vi "TDT ET-Send Command.vi"(0 "TCP":T1, 2 "Command":T2, 7 "Param (int)":i32, 9 "Timeout (ms)":i32=5000, 11 "error in (no error)":errorcluster) -> (4 "TCP Thru":T1, 10 "Return Value":i32, 15 "error out":errorcluster)   [LabVIEW 2020]
uses:
  Utility VIs/Type Defs/TCP Params.ctl
  TDT ET-Command Enum.ctl
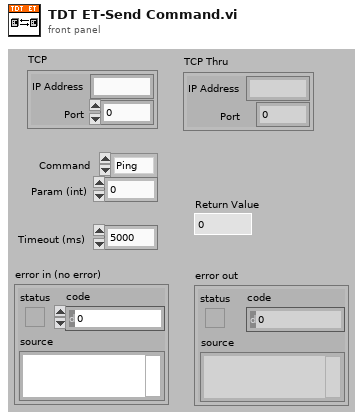
[diagram p1: front panel]
types:
  T1 = typedef "TCP Params.ctl" = cluster{"IP Address":string, "Port":i32}
  T2 = typedef "TDT ET-Command Enum.ctl" = enum16{"Ping", "Start", "Stop", "NewBlock"}
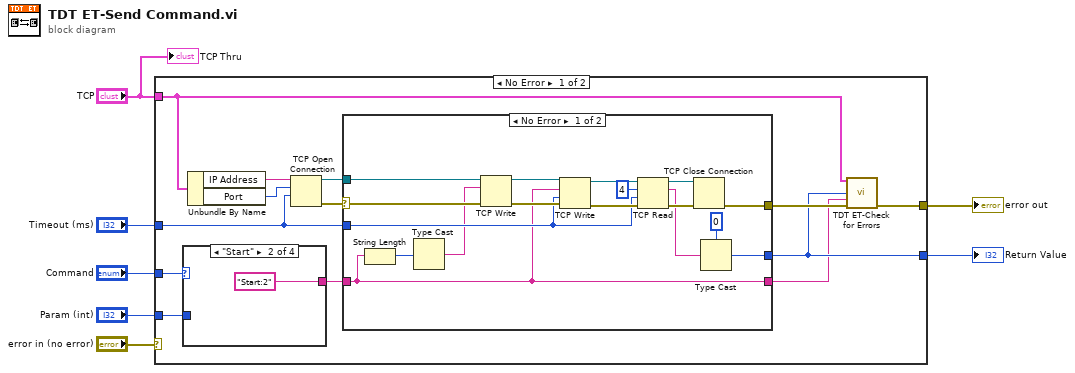
[diagram p0: block diagram]
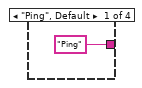
[diagram p2: hidden frame]
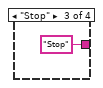
[diagram p3: hidden frame]
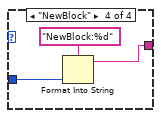
[diagram p4: hidden frame]
diagram:
  n1 = case shown="No Error" "error in (no error)" {
    selector: "error in (no error)" -> [_ w46]
    tunnel: [w11 w46] -> w6
    tunnel: "TCP" -> [w10 _]
    tunnel: "Timeout (ms)" -> [w15 _]
    tunnel: "Command" -> [w17 _]
    tunnel: [w9 _] -> w3
    tunnel: "Param (int)" -> [w12 _]
    frame No Error {
      n2 = case shown="\"Start\"" w17 {
        tunnel: ["Ping" "Start:2" "Stop" w25] -> w16
        tunnel: w12 -> [_ _ _ w24]
        frame "Ping", Default {
        }
        frame "Start" {
        }
        frame "Stop" {
        }
        frame "NewBlock" {
          n3 = Format Into String(format string="NewBlock:%d", w24) -> (resulting string=w25:string)  [unwired: 2 in, 1 out]
        }
      }
      n4 = Unbundle By Name(w10) -> ("IP Address"=w13:string, "Port"=w20:i32)
      n5 = TCP Open Connection(address=w13, remote port or service name=w20, timeout ms (60000)=w15) -> (connection ID=w18:refnum<k5>, error out=w19:errorcluster)  [unwired: 2 in]
      n6 = case shown="No Error" w19 {
        selector: w19 -> [w32 w44]
        tunnel: w18 -> [w31 _]
        tunnel: w16 -> [w27 w45]
        tunnel: w15 -> [w39 _]
        tunnel: [w36 w44] -> w14
        tunnel: [w33 _] -> w9
        tunnel: [w27 w45] -> w8
        frame No Error {
          n7 = String Length(string=w27) -> (length=w29:i32)
          n8 = Type Cast(x=w29) -> (*(type *) &x=w28:string)  [unwired: 1 in]
          n9 = TCP Write(connection ID=w31, data in=w28, error in (no error)=w32) -> (connection ID out=w30:refnum<k5>, error out=w43:errorcluster)  [unwired: 1 in, 1 out]
          n10 = TCP Write(connection ID=w30, data in=w27, error in (no error)=w43, 9:w39) -> (connection ID out=w41:refnum<k5>, error out=w42:errorcluster)  [unwired: 1 out]
          n11 = TCP Read(connection ID=w41, bytes to read=4, error in (no error)=w42, 9:w39) -> (connection ID out=w37:refnum<k5>, data out=w35:string, error out=w38:errorcluster)  [unwired: 1 in]
          n12 = TCP Close Connection(connection ID=w37, error in (no error)=w38) -> (error out=w36:errorcluster)  [unwired: 1 in, 1 out]
          n13 = Type Cast(type=0, x=w35) -> (*(type *) &x=w33:i32)
        }
        frame Error {
        }
      }
      n14 = call "TDT ET-Check for Errors.vi"("TCP"=w10, "TCP return value"=w9, "Command"=w8, "error in (no error)"=w14) -> ("error out"=w11:errorcluster)  [unwired: 10 in, 1 out]
    }
    frame Error {
    }
  }
  "error out" <- w6
  "Return Value" <- w3
  "TCP Thru" <- "TCP"
